vi "immediate.vi"(7 "Description":string, 8 "Command Info In":T1, 9 "tilt":dbl, 10 "intake":dbl, 11 "shooter":dbl) -> (0 "Command Info Out":T1)   [LabVIEW 2017]
doc: "This template is useful for immediate subsystem actions that do not need deadband filtering\n\nBe sure to right-click and select New from Template and save with a new command name."
uses:
  <vilib>/Rock Robotics/WPI/Framework/Command Status Info.ctl
  <vilib>/Rock Robotics/WPI/Framework/Completion Status.ctl
  <vilib>/Rock Robotics/WPI/Framework/Completion Notifier.ctl
  Implementation/Shooter Setpoints.ctl
  Implementation/Shooter Operations.ctl
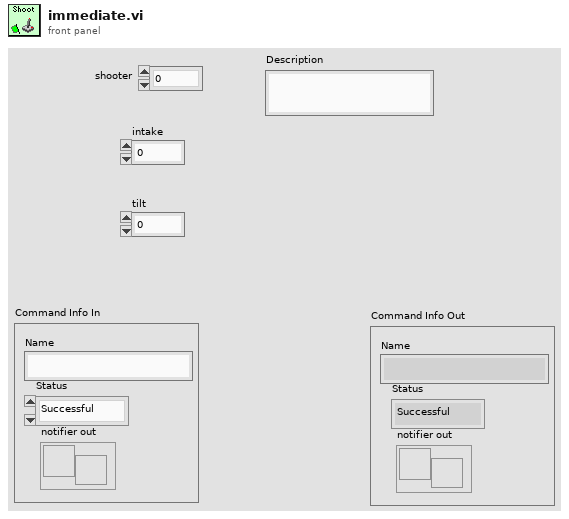
[diagram p1: front panel]
types:
  T1 = typedef "Command Status Info.ctl" = cluster{"Name":string, "Status":T2, "notifier out":T3}
  T2 = typedef "Completion Status.ctl" = enum16{"Successful", "Aborted", "Incomplete"}
  T3 = typedef "Completion Notifier.ctl" = refnum<notifier>
  T4 = typedef "Shooter Operations.ctl" = enum16{"Reserve", "Read Current", "Immediate", "Shoot"}
  T5 = typedef "Shooter Setpoints.ctl" = cluster{"Operation":T4, "shooterSetpoint":dbl, "Duration":dbl, "intakeste":dbl, "tilt":dbl}
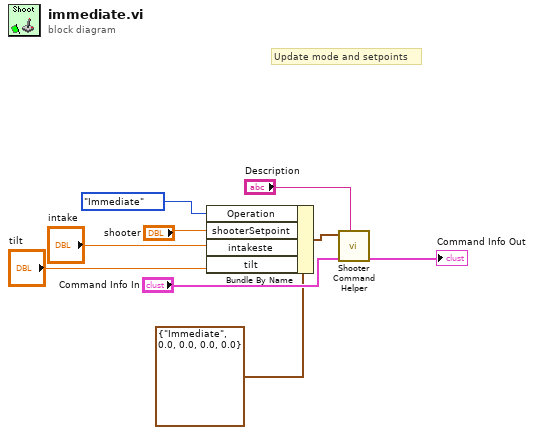
[diagram p0: block diagram]
diagram:
  # "Update mode and setpoints"
  n1 = Bundle By Name(cluster=T5 {"Operation"=enum."Immediate", "shooterSetpoint"=0.0, "Duration"=0.0, "intakeste"=0.0, "tilt"=0.0} ("SubSystem Data"), "Operation"=Shooter_Operations."Immediate", "shooterSetpoint"="shooter", "intakeste"="intake", "tilt"="tilt") -> (w4:T5)
  n2 = call "Shooter Command Helper.vi"("Description"="Description", "Command Info In"="Command Info In", "SubSystem Data"=w4) -> ("Command Info Out"=→"Command Info Out":T1)  [unwired: 6 in, 2 out]
